vi "Untitled 2 (SubVI).vi"(7 "error in":errorcluster, 9 "Data":T1, 10 "CRDS in":refnum<class "CRDS.lvclass">=refnum) -> (0 "error out":errorcluster, 3 "CRDS out":refnum<class "CRDS.lvclass">)   [LabVIEW 2014, in "CRDS.lvclass"]
uses:
  CRDS.lvclass
  Cell/hkParam Ctl.ctl
  Data/Cell/CRDS Cell Data.lvclass
  Cell/CRDS Cell.lvclass
  Data/Main/CRDS Data.lvclass
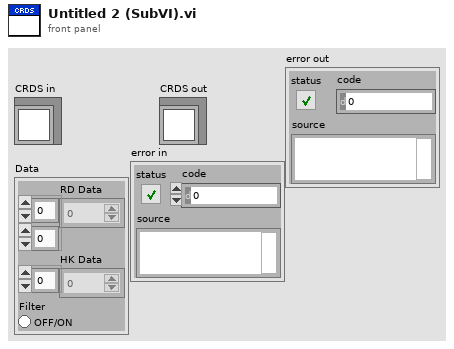
[diagram p1: front panel]
types:
  T1 = cluster{"RD Data":dbl[][], "HK Data":dbl[], "Filter":bool}
  T2 = typedef "CRDS Lib.lvlib/CRDS Cell Data.lvclass/hkParam Ctl.ctl" = cluster{"rhDilFac":sgl, "Q":sgl, "Tmean":sgl, "extDilFac":sgl, "rhCell":sgl, "P":sgl, "T":sgl}
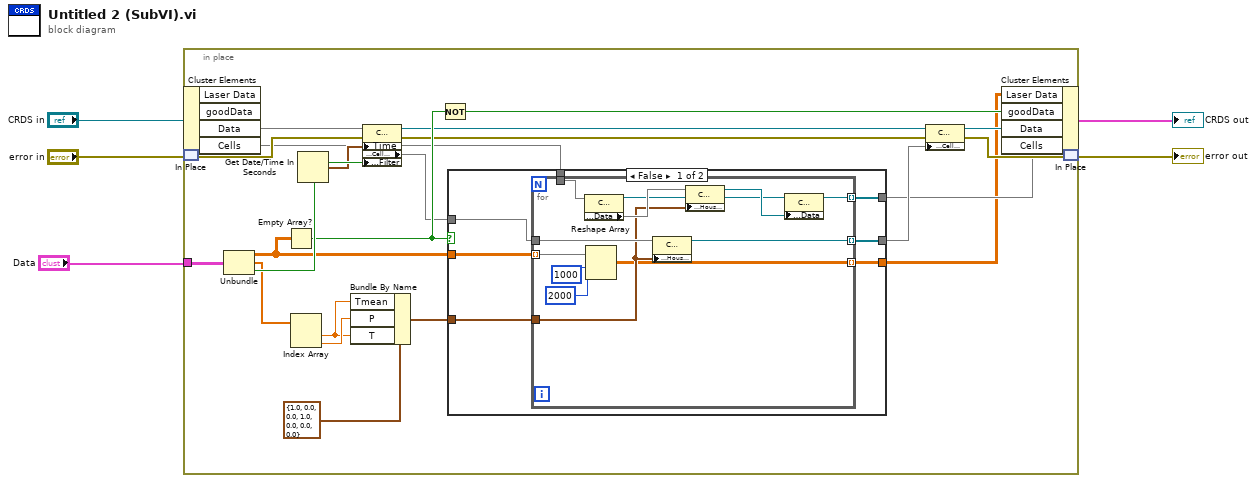
[diagram p0: block diagram]
diagram:
  n1 = in-place {
    in-place-border: "Data" -> [w20]
    n2 = in-place-cluster #1("CRDS in") -> ("Data"=w16, "Cells"=w8)  [unwired: 2 out]
    n3 = in-place-match #2("error in") -> (w14:errorcluster)
    n4 = Unbundle(w20) -> ("RD Data"=w9:dbl[][], "HK Data"=w21:dbl[], "Filter"=w27:bool)
    n5 = Empty Array?(array=w9) -> (empty?=w26:bool)
    n6 = Index Array(array=w21) -> (element #1=w23:dbl, element #2=w24:dbl)  [unwired: 2 in]
    n7 = Get Date/Time In Seconds() -> (seconds since 1Jan1904=w18:timestamp)
    n8 = Bundle By Name(cluster=T2 {"rhDilFac"=1.0, "Q"=0.0, "Tmean"=0.0, "extDilFac"=1.0, "rhCell"=0.0, "P"=0.0, "T"=0.0} ("Housekeeping"), "Tmean"=w23, "P"=w24, "T"=w23) -> (w25:T2)
    n9 = property class="CRDS Data.lvclass"(reference=w16, error in=w14, "Time"=w18, "Accessors:Filter"=w27) -> (reference out=w19:refnum<class "CRDS Data.lvclass">, error out=w17:errorcluster, "Accessors:Cell Data"=w10)
    n10 = Not(x=w26) -> (.not. x?=w12:bool)
    n11 = case shown="False" w26 {
      tunnel: w10 -> [w34 w48]
      tunnel: w25 -> [w33 _]
      tunnel: [w32 w48] -> w11
      tunnel: w9 -> [w31 _]
      tunnel: w8 -> [w30 w47]
      tunnel: [w29 w47] -> w7
      tunnel: [w28 _] -> w6
      frame False {
        n12 = for {
          tunnel: w34 -> [w46]
          tunnel: w31 -> [w36] mode=indexing
          tunnel: [w43] -> w32 mode=indexing
          tunnel: w33 -> [w40]
          tunnel: w30 -> [w42]
          tunnel: [w37] -> w29 mode=indexing
          tunnel: [w35] -> w28 mode=indexing
          n13 = property class="CRDS Cell.lvclass"(reference=w42) -> (reference out=w38:refnum<class "CRDS Cell.lvclass">, "Data Access:Data"=w41)  [unwired: 1 in, 1 out]
          n14 = Reshape Array(w36, 1000 ("dimension size"), 2000 ("dimension size")) -> (w35:dbl[][])
          n15 = property class="CRDS Cell Data.lvclass"(reference=w46, "Data Access:Housekeeping"=w40) -> (reference out=w43:refnum<class "CRDS Cell Data.lvclass">)  [unwired: 1 in, 1 out]
          n16 = property class="CRDS Cell Data.lvclass"(reference=w41, "Data Access:Housekeeping"=w40) -> (reference out=w39:refnum<class "CRDS Cell Data.lvclass">)  [unwired: 1 in, 1 out]
          n17 = property class="CRDS Cell.lvclass"(reference=w38, "Data Access:Data"=w39) -> (reference out=w37:refnum<class "CRDS Cell.lvclass">)  [unwired: 1 in, 1 out]
        }
      }
      frame True {
      }
    }
    n18 = property class="CRDS Data.lvclass"(reference=w19, error in=w17, "Accessors:Cell Data"=w11) -> (reference out=w15:refnum<class "CRDS Data.lvclass">, error out=w13:errorcluster)
    n19 = in-place-cluster #1("Laser Data"=w6, "goodData"=w12, "Data"=w15, "Cells"=w7) -> (→"CRDS out":cluster{})
    n20 = in-place-match #2(w13) -> (→"error out":errorcluster)
  }
